vi "Read MVIName.vi"(8 "error in (no error)":errorcluster, 11 "MB Param in":refnum<class "MB Param.lvclass">) -> (0 "error out":errorcluster, 2 "MVIName":string, 3 "MB Param out":refnum<class "MB Param.lvclass">)   [LabVIEW 2021, in "MBParam.lvlib" / "MB Param.lvclass"]
uses:
  MB Param.lvclass
  MB Param.lvclass/MB Param.ctl
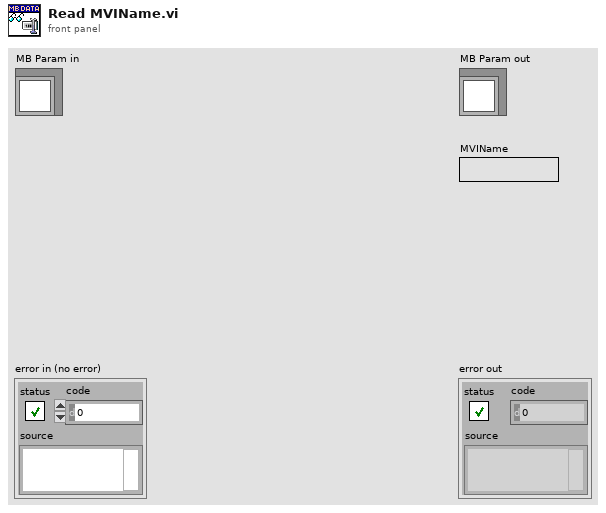
[diagram p1: front panel]
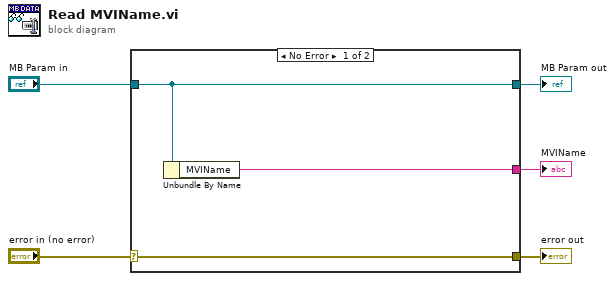
[diagram p0: block diagram]
diagram:
  n1 = case shown="No Error" "error in (no error)" {
    selector: "error in (no error)" -> [w8 w9]
    tunnel: [w8 w9] -> w4
    tunnel: [w7 w10] -> w2
    tunnel: "MB Param in" -> [w7 w10]
    tunnel: [w6 _] -> w1
    frame No Error {
      n2 = Unbundle By Name(w7) -> ("MVIName"=w6:string)
    }
    frame Error {
    }
  }
  "error out" <- w4
  "MB Param out" <- w2
  "MVIName" <- w1
